vi "simplePID Memory Read.vi"(1 "channel (0)":u8, 3 "Input Selector":u8) -> (4 "memory out":refnum<k21>="Data", 15 "state out":T1)   [LabVIEW 2020]
uses:
  <vilib>/rvi/Analysis/control/PID/Typedef/niFpgaPID_PIDState.ctl
  <vilib>/rvi/DataTransferAndStorage/Container/Common/niFpgaContainerGetUniqueNameForEmu.vi
  <vilib>/rvi/DataTransferAndStorage/Container/Common/niFpgaContainerSetEmuInfo.vi
  <vilib>/rvi/eio/common/nirviEmuReportErrorAndStop.vi
  <vilib>/rvi/DataTransferAndStorage/Container/Common/niFpgaContainerExecOnDevCompGetState.vi
  <vilib>/rvi/Emulation/niFpgaEmulationIsFPGAContextNoSignature.vi
  <vilib>/rvi/Emulation/niFpgaProcessEmulError.vi
  <vilib>/rvi/Emulation/niFpgaSctlEmulationGetInTimedLoop.vi
  <vilib>/rvi/errors/nirviReportUnexpectedCaseInternalError (U32).vi
  <vilib>/rvi/Memory/Memory_Emulation/niFpgaMemoryEmulationCacheClearOnFirstRun.vi
  <vilib>/rvi/Memory/Memory_Emulation/nirvimemoryEmulationManagerCache_MakeExclusive.vi
  <vilib>/rvi/Memory/Memory_Emulation/niFpgaMemoryEmulationValidateCache.vi
  <vilib>/rvi/Memory/Memory_Emulation/nirvimemoryEmulationManagerCache_InsertValue.vi
  <vilib>/Utility/error.llb/Clear Errors.vi
  <vilib>/rvi/Memory/Memory_Emulation/nirvimemoryEmulationManagerCache_ReleaseExclusive.vi
  <vilib>/rvi/Memory/Memory_Emulation/nirvimemoryEmulationManagerCache_GetValue.vi
  <vilib>/rvi/Memory/Memory_Emulation/nirvimemoryEmulationManagerCache_SetValue.vi
  <vilib>/rvi/Emulation/niFpgaSctlEmulationResourceMgr.vi
  <vilib>/rvi/LocalResourceManager/LocalResourceManager.xnode
  <vilib>/rvi/DataTransferAndStorage/Container/XNode/niFpgaContainer.xnode
  <vilib>/rvi/Memory/Memory_Emulation/niFpgaMemoryEmulationRefIn.vi
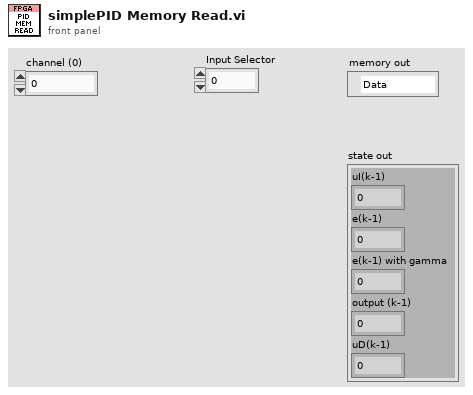
[diagram p1: front panel]
types:
  T1 = typedef "niFpgaPID_PIDState.ctl" = cluster{"uI(k-1)":sgl, "e(k-1)":sgl, "e(k-1) with gamma":sgl, "output (k-1)":sgl, "uD(k-1)":sgl}
  T2 = cluster{"data 1":sgl, "data 2":sgl, "data 3":sgl, "data 4":sgl}
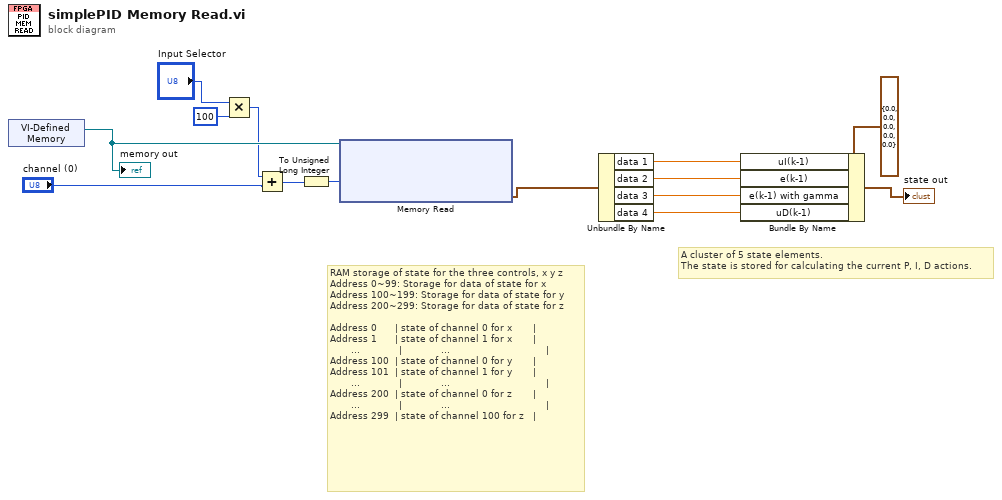
[diagram p0: block diagram]
diagram:
  # "RAM storage of state for the three controls, x y z\nAddress 0~99: Storage for data of state for x\nAddress 100~199: Storage for data of state for y\nAddress 200~299: Storage for data of state for z \n                                                                        \nAddress 0      | state of channel 0 for x       | \nAddress 1      | state of channel 1 for x       | \n       ...             |             ...                                |\nAddress 100  | state of channel 0 for y       | \nAddress 101  | state of channel 1 for y       | \n       ...             |             ...                                |\nAddress 200  | state of channel 0 for z       | \n       ...             |             ...                                |\nAddress 299  | state of channel 100 for z   |"
  # "A cluster of 5 state elements.\nThe state is stored for calculating the current P, I, D actions."
  n1 = xnode "VI-Defined Memory"() -> ("Memory Out"=w6:refnum<k21>)
  "memory out" <- w6
  n2 = Multiply(x="Input Selector", y=u8 100) -> (x*y=w4:u8)
  n3 = Add(x=w4, y="channel (0)") -> (x+y=w1:u8)
  n4 = To Unsigned Long Integer(number=w1) -> (unsigned 32bit integer=w8:u32)
  n5 = xnode ("Memory Read")("Address"=w8, "Memory In"=w6) -> ("Data"=w7:T2)  [unwired: 1 out]
  n6 = Unbundle By Name(w7) -> ("data 1"=w9:sgl, "data 2"=w10:sgl, "data 3"=w11:sgl, "data 4"=w12:sgl)
  n7 = Bundle By Name(cluster=T1 {"uI(k-1)"=0.0, "e(k-1)"=0.0, "e(k-1) with gamma"=0.0, "output (k-1)"=0.0, "uD(k-1)"=0.0} ("state out"), "uI(k-1)"=w9, "e(k-1)"=w10, "e(k-1) with gamma"=w11, "uD(k-1)"=w12) -> (→"state out":T1)
